vi "Generate_Waveforms.vi"(8 "error in (no error)":errorcluster, 11 "Generator":refnum<class "Generator.lvclass">) -> (0 "error out":errorcluster, 1 "phase out":dbl[](array[numeric]), 2 "AO Array":waveform(dbl)[](array[waveform]), 3 "Generator":refnum<class "Generator.lvclass">)   [LabVIEW 2016, in "Generator.lvclass"]
uses:
  Generator.lvclass
  Generator.lvclass/Generator.ctl
  <vilib>/measure/NI_MABase.lvlib
panel:
  in  "display graphs?":bool
  out "phase Chart":dbl[][](graph)
  out "Waveform Graph":waveform(dbl)[](graph)
  out "Numeric":i32
  # "if phase = 0, waveform is same as revious?"
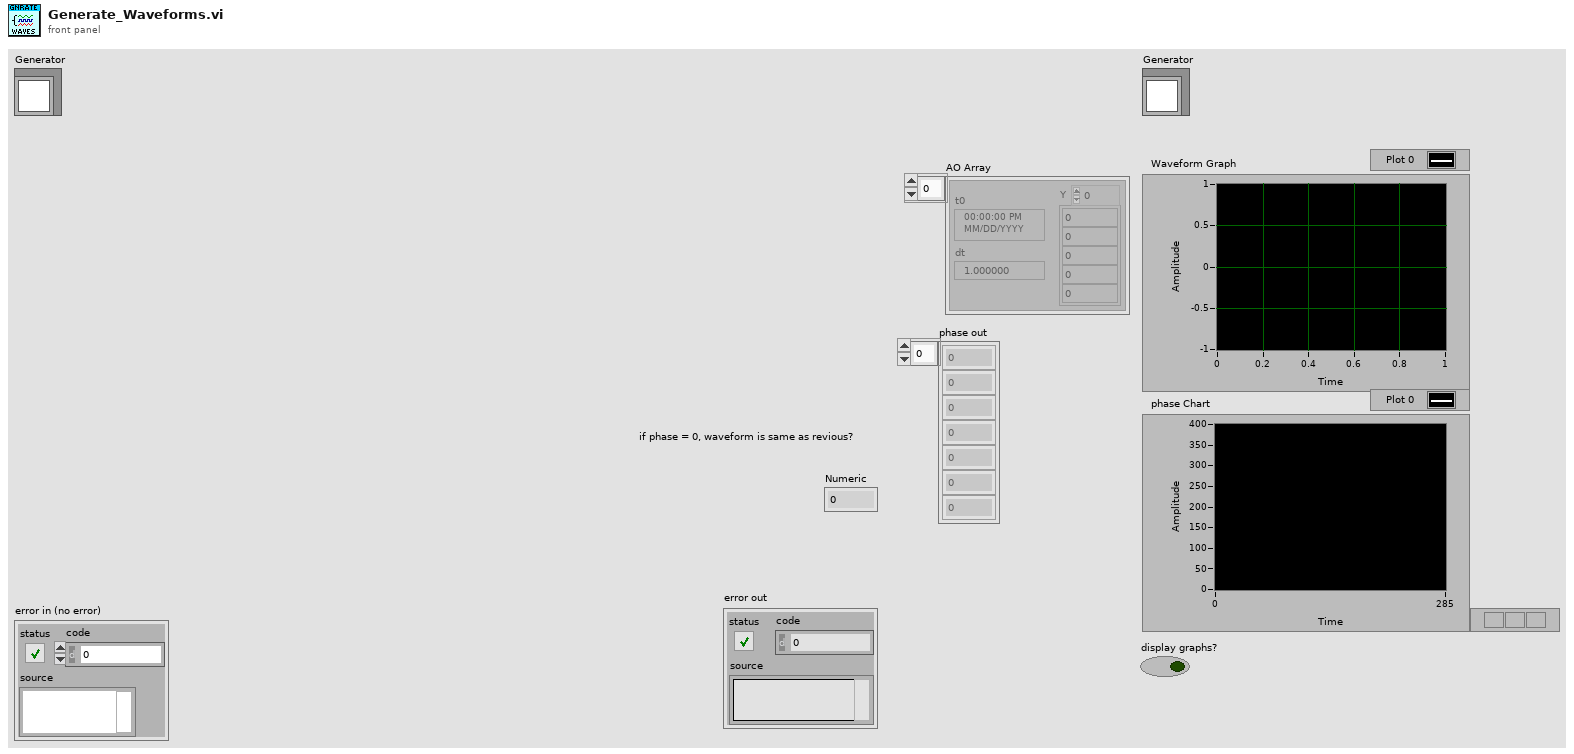
[diagram p1: front panel]
types:
  T1 = typedef "Generator.lvclass/PrivateEvents--Generator.configGenerator.ctl" = cluster{"A (V)":dbl, "DC (V)":dbl, "f (Hz)":dbl, "phi (deg)":dbl, "signal type":enum16{"Sine Wave", "Triangle Wave", "Square Wave", "Sawtooth Wave"}}[]
  T2 = typedef "Generator.lvclass/PrivateEvents--Generator.resetGenerator.ctl" = bool
  T3 = typedef "Generator.lvclass/PrivateEvents--Generator.configSampling.ctl" = cluster{"Fs":dbl, "#s":dbl}
  T4 = enum16{"Sine Wave", "Triangle Wave", "Square Wave", "Sawtooth Wave"}
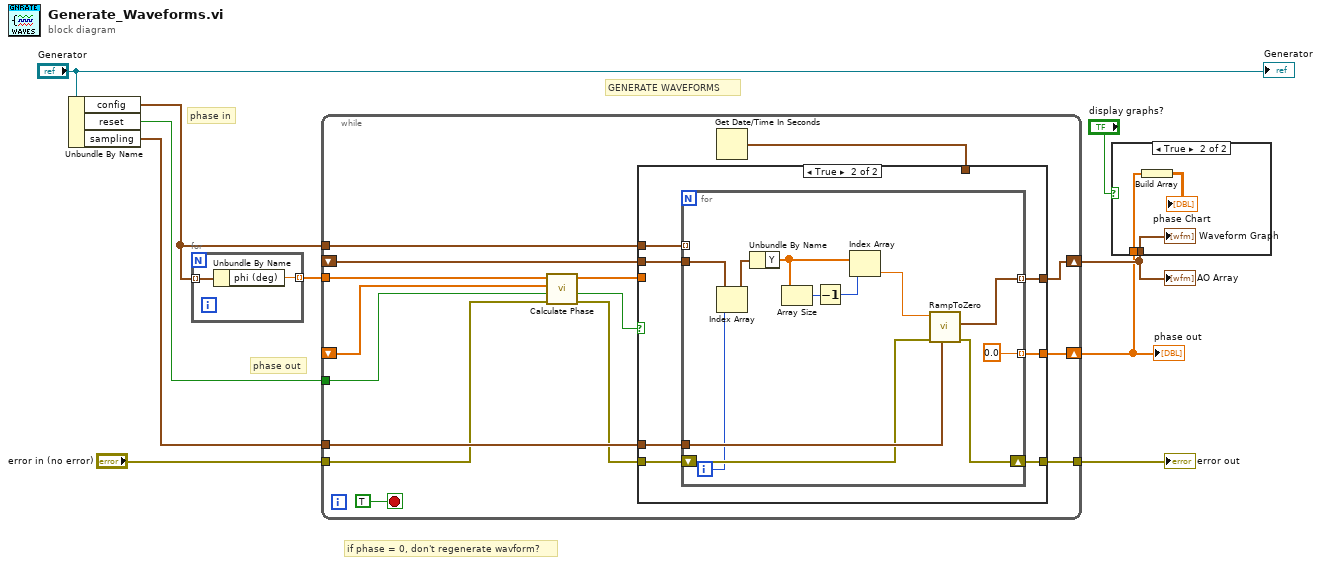
[diagram p0: block diagram]
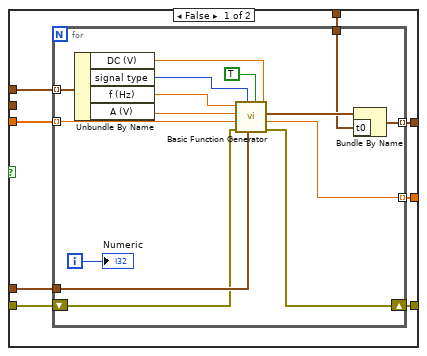
[diagram p3: hidden frame]
diagram:
  # "phase out"
  # "phase in"
  # "if phase = 0, don't regenerate wavform?"
  # "GENERATE WAVEFORMS"
  n1 = Unbundle By Name("Generator") -> ("config"=w4:T1, "reset"=w3:T2, "sampling"=w2:T3)
  n2 = for {
    tunnel: w4 -> [w12] mode=indexing
    tunnel: [w11] -> w6 mode=indexing
    n3 = Unbundle By Name(w12) -> ("phi (deg)"=w11:dbl)
  }
  n4 = while {
    tunnel: w2 -> [w24]
    tunnel: w6 -> [w22]
    shift-right: [w25] -> w7
    shift-left: _ -> [w21]
    tunnel: w3 -> [w20]
    tunnel: "error in (no error)" -> [w16]
    tunnel: [w17] -> w9
    tunnel: w4 -> [w19]
    shift-right: [w27] -> w8
    shift-left: _ -> [w13]
    stop <- TRUE stop-if-true
    n5 = call "Calculate Phase.vi"("error in (no error)"=w16, "reset phase"=w20, "phase out"=w21, "config phase"=w22) -> ("error out"=w18:errorcluster, "reset?"=w14:bool, "adjusted phase"=w23:dbl[])  [unwired: 5 in]
    n6 = Get Date/Time In Seconds() -> (seconds since 1Jan1904=w15:timestamp)
    n7 = case shown="True" w14 {
      tunnel: [w35 w52] -> w27
      tunnel: [w34 w57] -> w25
      tunnel: w24 -> [w33 w55]
      tunnel: w23 -> [w32 _]
      tunnel: w19 -> [w31 w51]
      tunnel: w18 -> [w30 w54]
      tunnel: [w29 w53] -> w17
      tunnel: w15 -> [w28 _]
      tunnel: w13 -> [_ w56]
      frame False {
        n8 = for {
          tunnel: [w47] -> w35 mode=indexing
          tunnel: w33 -> [w45]
          tunnel: [w46] -> w34 mode=indexing
          tunnel: w32 -> [w44] mode=indexing
          tunnel: w31 -> [w43] mode=indexing
          shift-right: [w37] -> w29
          shift-left: w30 -> [w38]
          tunnel: w28 -> [w36]
          i -> [w49]
          n9 = Unbundle By Name(w43) -> ("DC (V)"=w40:dbl, "signal type"=w39:T4, "f (Hz)"=w41:dbl, "A (V)"=w42:dbl)
          n10 = call <vilib>:"Basic Function Generator.vi"("offset"=w40, "reset signal"=TRUE, "sampling info"=w45, "signal type"=w39, "error in (no error)"=w38, "phase"=w44, "amplitude"=w42, "frequency"=w41) -> ("error out"=w37:errorcluster, "phase out"=w46:dbl, "signal out"=w50:waveform(dbl))  [unwired: 1 in]
          n11 = Bundle By Name(cluster=w50, "t0"=w36) -> (w47:waveform(dbl))
          "Numeric" <- w49
        }
      }
      frame True {
        n12 = for {
          tunnel: [0.0] -> w57 mode=indexing
          tunnel: w56 -> [w60]
          tunnel: w55 -> [w64]
          tunnel: [w61] -> w52 mode=indexing
          shift-right: [w62] -> w53
          shift-left: w54 -> [w63]
          tunnel: w51 -> [_] mode=indexing
          i -> [w59]
          n13 = Index Array(array=w60, index=w59) -> (element=w58:waveform(dbl))
          n14 = Unbundle By Name(w58) -> ("Y"=w68:dbl[])
          n15 = Array Size(array=w68) -> (size(s)=w67:i32)
          n16 = Decrement(x=w67) -> (x-1=w66:i32)
          n17 = Index Array(array=w68, index=w66) -> (element=w65:dbl)
          n18 = call "RampToZero.vi"("sampling info"=w64, "error in (no error)"=w63, "starting value"=w65) -> ("error out"=w62:errorcluster, "Waveform Graph"=w61:waveform(dbl))  [unwired: 7 in]
        }
      }
    }
  }
  "AO Array" <- w8
  "error out" <- w9
  "phase out" <- w7
  n19 = case shown="True" "display graphs?" {
    tunnel: w8 -> [_ w72]
    tunnel: w7 -> [_ w71]
    frame False {
    }
    frame True {
      n20 = Build Array(w71) -> (→"phase Chart":dbl[][])
      "Waveform Graph" <- w72
    }
  }
  "Generator" <- "Generator"
